vi "Configure LPC.vi"(6 "front-panel controls":enum16{"enabled", "disabled"}(ring), 7 "power":dbl[unit]=0.005, 8 "error in (no error)":errorcluster, 9 "control mode":T1(ring), 10 "wavelength":dbl[unit]=8.300000000000001e-07, 11 "VISA resource name":refnum<visa-resource-name>="GPIB0::8::INSTR") -> (0 "error out":errorcluster, 3 "VISA resource name out":refnum<visa-resource-name>)   [LabVIEW 2009, in "Laser Power Controller.lvclass"]
doc: "Configures the most important (to us) settings for the LPC (laser power controller)."
uses:
  Laser Power Controller.lvclass
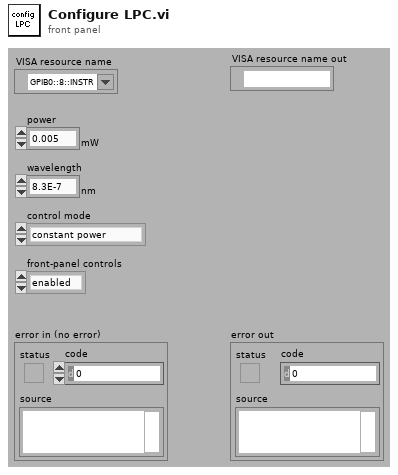
[diagram p1: front panel]
types:
  T1 = enum16{"constant power", "constant transmission"}
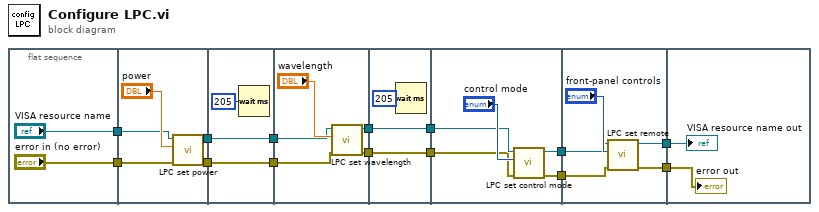
[diagram p0: block diagram]
diagram:
  n1 = flat-sequence {
    tunnel: ["VISA resource name"] -> w14
    tunnel: ["error in (no error)"] -> w13
    tunnel: w14 -> [w20]
    tunnel: w13 -> [w19]
    tunnel: [w18] -> w8
    tunnel: [w17] -> w6
    tunnel: w8 -> [w24]
    tunnel: [w24] -> w7
    tunnel: w6 -> [w23]
    tunnel: [w23] -> w5
    tunnel: w7 -> [w28]
    tunnel: w5 -> [w27]
    tunnel: [w26] -> w4
    tunnel: [w25] -> w2
    tunnel: w4 -> [w32]
    tunnel: [w32] -> w3
    tunnel: w2 -> [w31]
    tunnel: [w31] -> w1
    tunnel: w3 -> [w36]
    tunnel: w1 -> [w35]
    tunnel: [w34] -> w12
    tunnel: [w33] -> w11
    tunnel: w12 -> [w41]
    tunnel: w11 -> [w40]
    tunnel: [w39] -> w10
    tunnel: [w38] -> w9
    tunnel: w10 -> [w44]
    tunnel: w9 -> [w43]
    frame #0 {
    }
    frame #1 {
      n2 = call "LPC set power.vi"("error in (no error)"=w19, "power"="power", "VISA resource name"=w20) -> ("error out"=w17:errorcluster, "VISA resource name out"=w18:refnum<visa-resource-name>)  [unwired: 7 out]
    }
    frame #2 {
      n3 = Wait (ms)(milliseconds to wait=u32 205) -> ()  [unwired: 1 out]
    }
    frame #3 {
      n4 = call "LPC set wavelength.vi"("error in (no error)"=w27, "wavelength"="wavelength", "VISA resource name"=w28) -> ("error out"=w25:errorcluster, "VISA resource name out"=w26:refnum<visa-resource-name>)  [unwired: 7 out]
    }
    frame #4 {
      n5 = Wait (ms)(milliseconds to wait=u32 205) -> ()  [unwired: 1 out]
    }
    frame #5 {
      n6 = call "LPC set control mode.vi"("error in (no error)"=w35, "control mode"="control mode", "VISA resource name"=w36) -> ("error out"=w33:errorcluster, "VISA resource name out"=w34:refnum<visa-resource-name>)  [unwired: 7 out]
    }
    frame #6 {
      n7 = call "LPC set remote.vi"("error in (no error)"=w40, "front-panel controls"="front-panel controls", "VISA resource name"=w41) -> ("error out"=w38:errorcluster, "VISA resource name out"=w39:refnum<visa-resource-name>)  [unwired: 7 out]
    }
    frame #7 {
      "VISA resource name out" <- w44
      "error out" <- w43
    }
  }
